vi "AMZ_S3_APIHLP_Parse AC List XML String from ACP.vi"(8 "error in (no error)":errorcluster, 11 "AccessControlPolicy":T1) -> (0 "error out":errorcluster, 3 "AccessControlList XML":string)   [LabVIEW 2015, in "LV Interface for Amazon S3.lvlib"]
uses:
  LV Interface for Amazon S3.lvlib
  Typedefs/AMZ_S3_API_AccessControlPolicy.ctl
  Typedefs/AMZ_S3_API_Owner.ctl
  Typedefs/AMZ_S3_API_Bucket ACL Permission.ctl
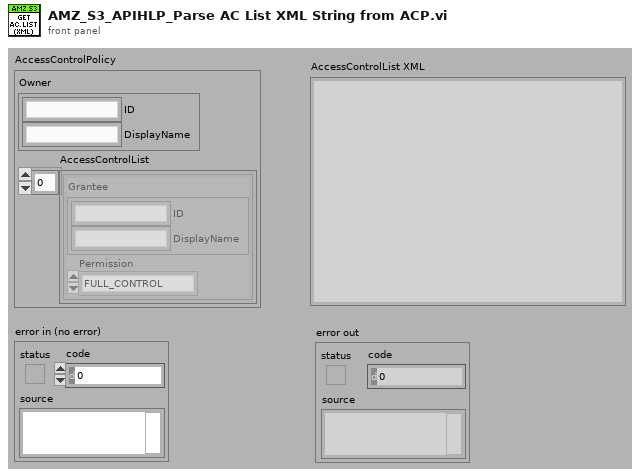
[diagram p1: front panel]
types:
  T1 = typedef "LV Interface for Amazon S3.lvlib/AMZ_S3_API_AccessControlPolicy.ctl" = cluster{"Owner":T2, "AccessControlList":cluster{"Grantee":T2, "Permission":T3}[]}
  T2 = typedef "LV Interface for Amazon S3.lvlib/AMZ_S3_API_Owner.ctl" = cluster{"ID":string, "DisplayName":string}
  T3 = typedef "LV Interface for Amazon S3.lvlib/AMZ_S3_API_Bucket ACL Permission.ctl" = enum16{"FULL_CONTROL", "WRITE", "WRITE_ACP", "READ", "READ_ACP"}
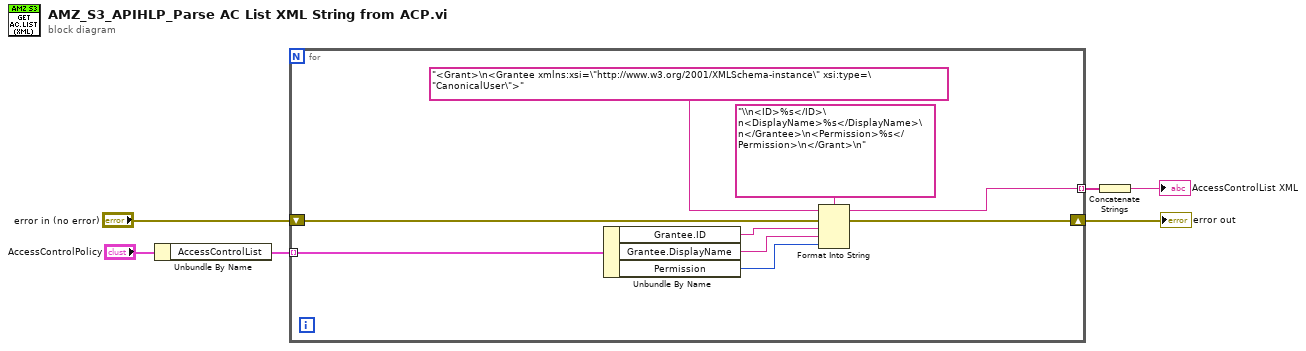
[diagram p0: block diagram]
diagram:
  n1 = Unbundle By Name("AccessControlPolicy") -> ("AccessControlList"=w5:cluster{"Grantee":T2, "Permission":T3}[])
  n2 = for {
    tunnel: w5 -> [w15] mode=indexing
    shift-right: [w8] -> w3
    shift-left: "error in (no error)" -> [w9]
    tunnel: [w7] -> w2 mode=indexing
    n3 = Unbundle By Name(w15) -> ("Grantee.ID"=w12:string, "Grantee.DisplayName"=w11:string, "Permission"=w10:T3)
    n4 = Format Into String(format string="\\n<ID>%s</ID>\n<DisplayName>%s</DisplayName>\n</Grantee>\n<Permission>%s</Permission>\n</Grant>\n", initial string="<Grant>\n<Grantee xmlns:xsi=\"http://www.w3.org/2001/XMLSchema-instance\" xsi:type=\"CanonicalUser\">", error in=w9, w12, w11, w10) -> (resulting string=w7:string, error out=w8:errorcluster)
  }
  "error out" <- w3
  n5 = Concatenate Strings(w2) -> (→"AccessControlList XML":string)
